vi "Get Enable.vi"(8 "error in (no error)":errorcluster, 11 "Fault-Injection_Boolean in":refnum<class "Fault-Injection_CEXT.lvclass">) -> (0 "error out":errorcluster, 2 "Enable?":bool, 3 "Fault-Injection_Boolean out":refnum<class "Fault-Injection_CEXT.lvclass">)   [LabVIEW 2021, in "Fault-Injection_CEXT.lvclass"]
uses:
  Fault-Injection_CEXT.lvclass
  Fault-Injection_CEXT.lvclass/Fault-Injection_CEXT.ctl
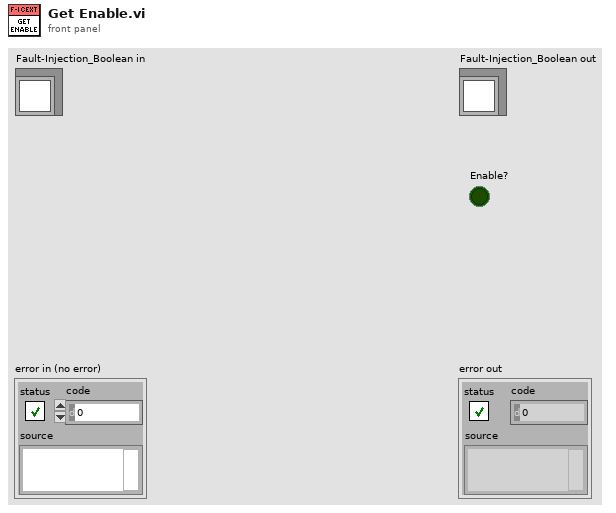
[diagram p1: front panel]
types:
  T1 = typedef "Fault-Injection_CEXT.lvclass/DVR Type.ctl" = cluster{"Enable":bool, "Injected Value":T2, "Value":T3}
  T2 = typedef "Fault-Injection_CEXT.lvclass/Value Type.ctl" = cxt
  T3 = typedef "Fault-Injection_CEXT.lvclass/Abs Class Type.ctl" = refnum<class "Abs_Complex Extended Float.lvclass">
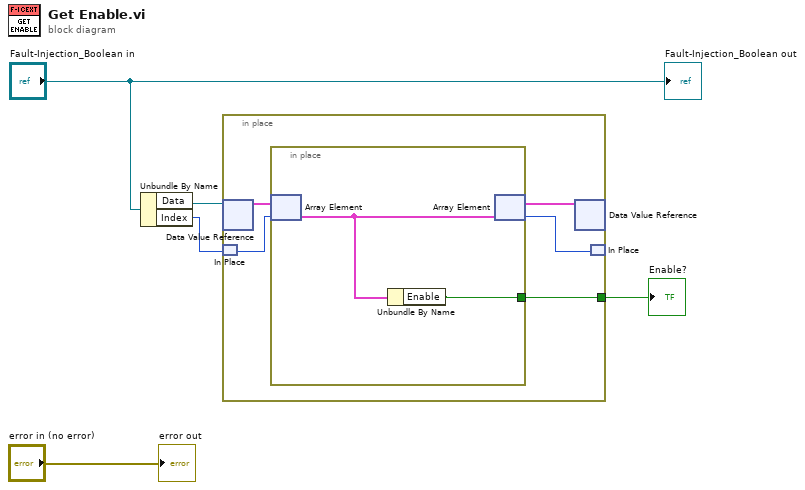
[diagram p0: block diagram]
diagram:
  n1 = Unbundle By Name("Fault-Injection_Boolean in") -> ("Data"=w4:refnum<data-value>, "Index"=w3:i32)
  n2 = in-place {
    in-place-border: [w6] -> w1
    n3 = in-place-dvr #1(w4) -> (w10:T1[])  [unwired: 1 out]
    n4 = in-place-match #2(w3) -> (w8:i32)
    n5 = in-place {
      in-place-border: [w11] -> w6
      n6 = in-place-array #3(w10, w8) -> (w12:T1)
      n7 = Unbundle By Name(w12) -> ("Enable"=w11:bool)
      n8 = in-place-array #3(w12) -> (w9:T1[], w7:i32)
    }
    n9 = in-place-dvr #1(w9) -> ()  [unwired: 2 out]
    n10 = in-place-match #2(w7) -> ()  [unwired: 1 out]
  }
  "Enable?" <- w1
  "error out" <- "error in (no error)"
  "Fault-Injection_Boolean out" <- "Fault-Injection_Boolean in"
